vi "ClusterToBSONDocument.vi"(8 "error in (no error)":errorcluster, 11 "Variant":variant) -> (0 "error out":errorcluster, 3 "tBSONDocument out":refnum<class "tBSONDocument.lvclass">)   [LabVIEW 2013, in "BSON.lvlib" / "tBSONDocument.lvclass"]
doc: "Converts simple LabVIEW clusters into a BSON document. The cluster must contain only basic types including numerics, timestamps, strings, paths, booleans, and clusters. Single dimension arrays of these types are also supported. There is limited analog waveform support although waveform attributes are not added to the document."
uses:
  tBSONDocument.lvclass
  status.ctl
  addI32Element.vi
  addI64Element.vi
  addDoubleElement.vi
  addBooleanElement.vi
  addStringElement.vi
  addTimestampElement.vi
  addDocumentElement.vi
  addI32[]Element.vi
  addI64[]Element.vi
  addDouble[]Element.vi
  addBoolean[]Element.vi
  addString[]Element.vi
  addTimestamp[]Element.vi
  addDocument[]Element.vi
  <vilib>/Utility/VariantDataType/VariantType.lvlib
  BSON.lvlib
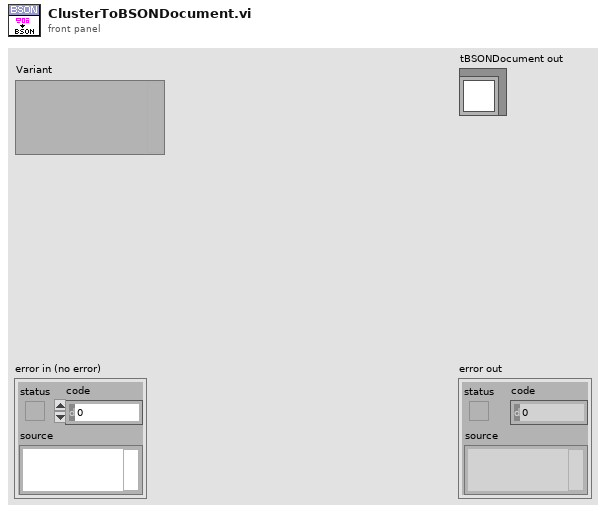
[diagram p1: front panel]
types:
  T1 = typedef "BSON.lvlib/status.ctl" = enum16{"Stream Corrupted or Ended Abruptly", "Incorrect Type In Stream", "ObjectID Invalid", "Method Not Implemented", "Invalid Name", "Invalid URI", "AutoReconnect", "Operation Failed", "Incorrectly Configured", "Cursor Not Found", "Timeout", "Invalid Type", "Empty Name", "Duplicate Name", "MD5Incorrect"}
  T2 = typedef "VariantType.lvlib/Type.ctl" = enum8{"Invalid Type", "Void", "I8", "I16", "I32", "I64", "U8", "U16", "U32", "U64", "Single Float", "Double Float", "Extended Float", "Single Complex", "Double Complex", "Extended Complex", "Enum U8", "Enum U16", "Enum U32", "Enum U64", "Single Float With Unit", "Double Float With Unit", "Extended Float With Unit", "Single Complex with Unit", "Double Complex with Unit", "Extended Complex with Unit", "Boolean", "String", "Path", "Picture", "Tag", "Array", "Cluster", "Variant", "LV Variant", "Waveform", "Timestamp", "Digital Waveform", "Digital Data", "ExpressData", "Refnum", "External Data", "VI", "Poly VI", "LabVIEW Class Instance", "Fixed Point"}
  T3 = typedef "VariantType.lvlib/MemoryInfo.ctl" = cluster{"Type":T4, "Size":u32}
  T4 = typedef "VariantType.lvlib/MemoryType.ctl" = enum16{"Variable", "Fixed", "Bounded"}
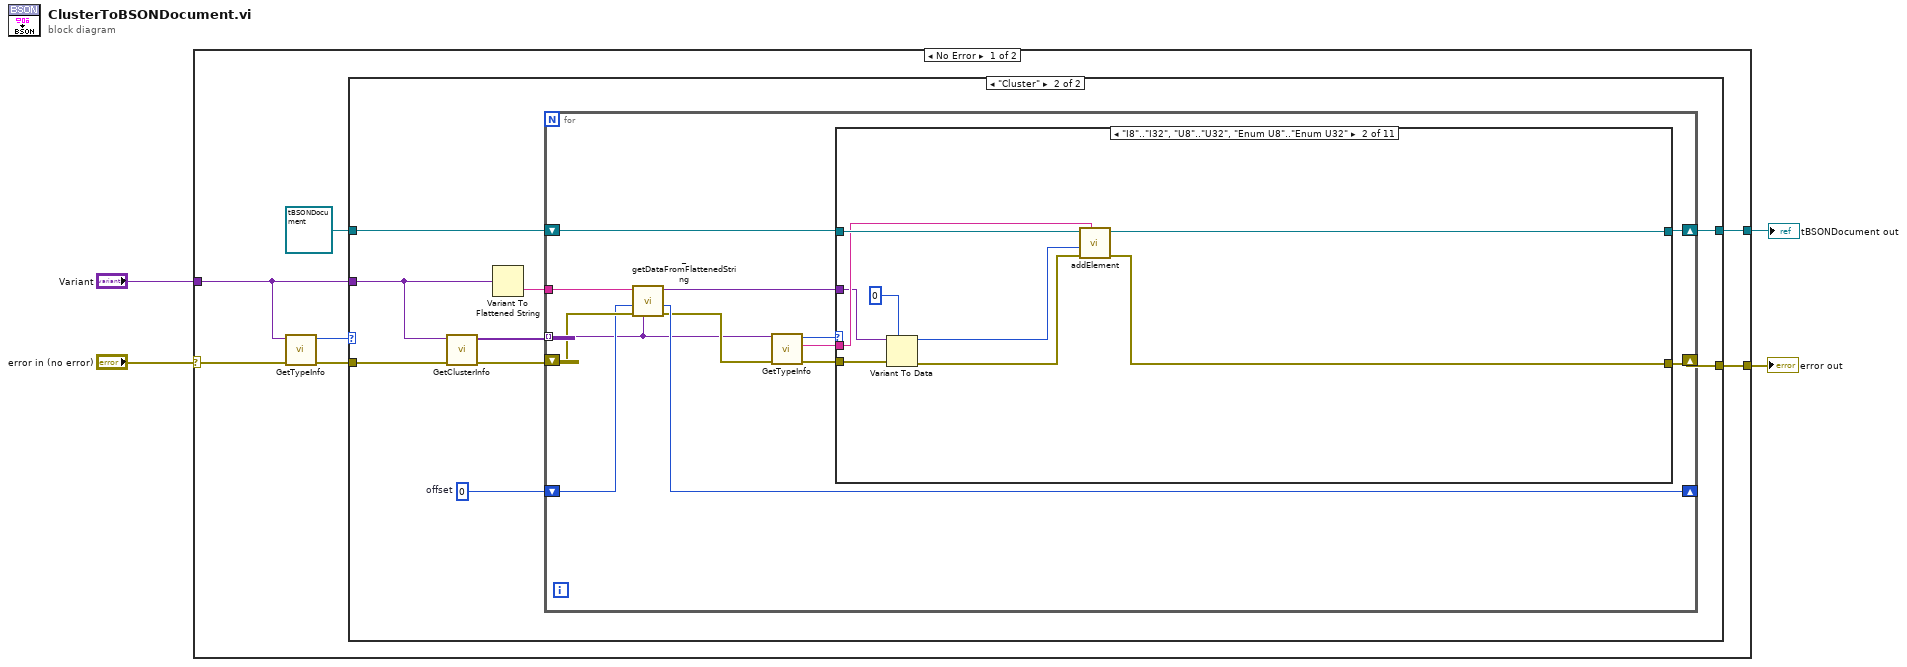
[diagram p0: block diagram]
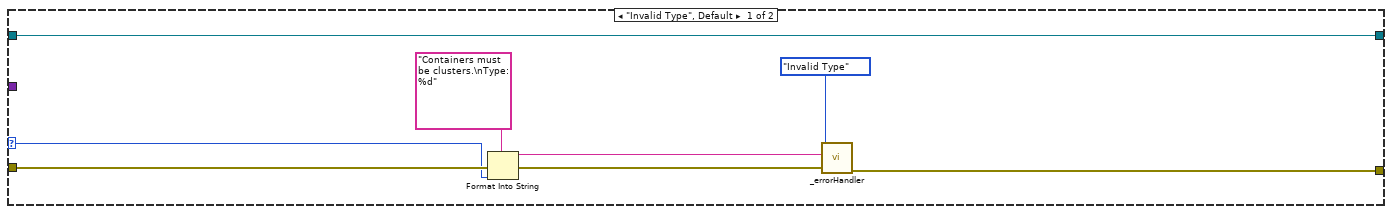
[diagram p2: hidden frame]
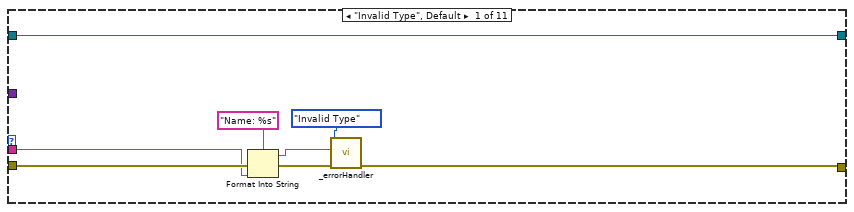
[diagram p3: hidden frame]
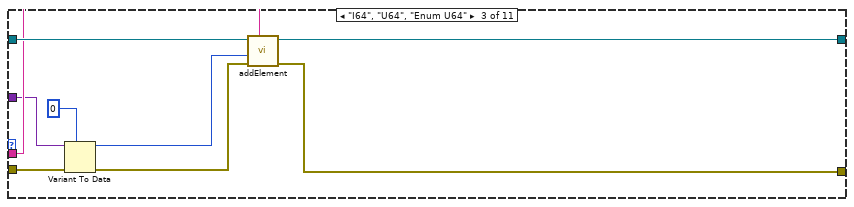
[diagram p4: hidden frame]
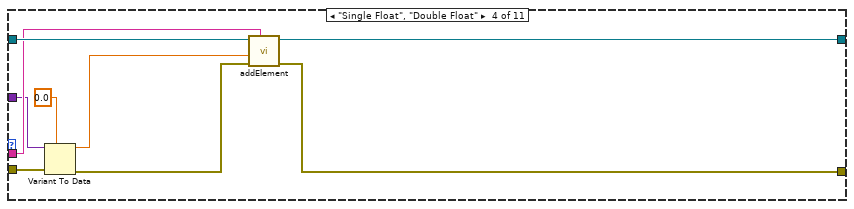
[diagram p5: hidden frame]
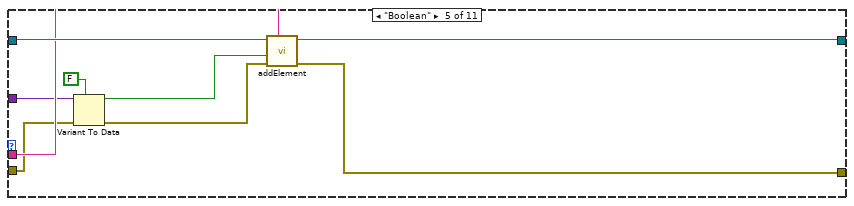
[diagram p6: hidden frame]
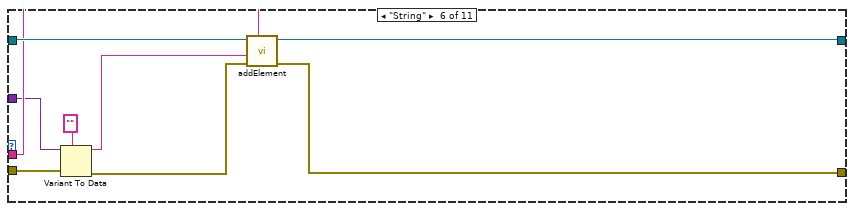
[diagram p7: hidden frame]
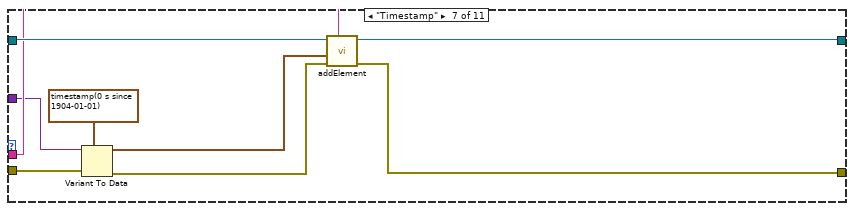
[diagram p8: hidden frame]
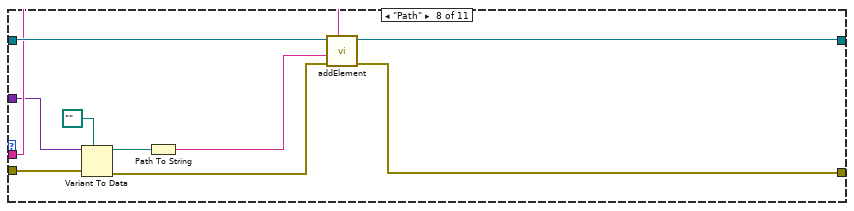
[diagram p9: hidden frame]
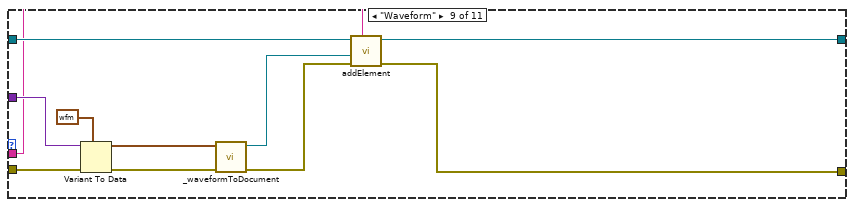
[diagram p10: hidden frame]
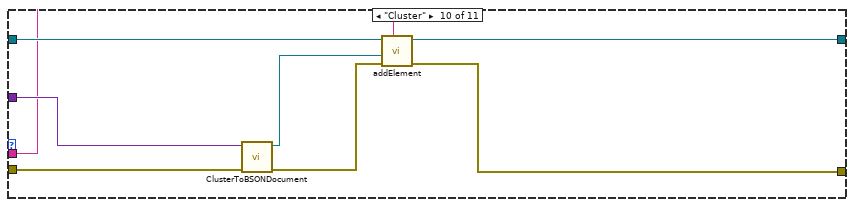
[diagram p11: hidden frame]
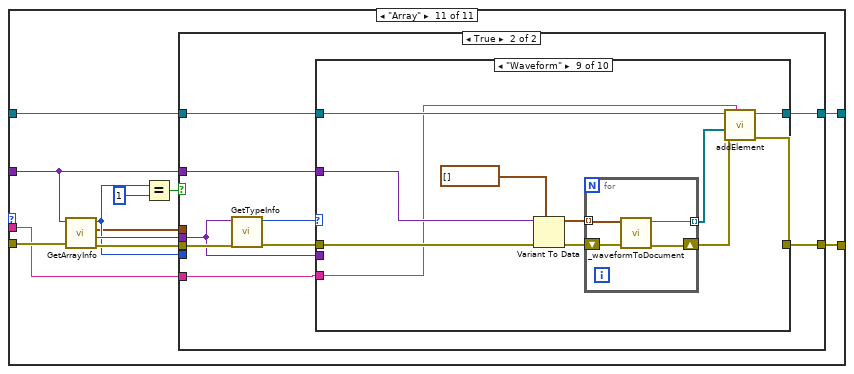
[diagram p12: hidden frame]
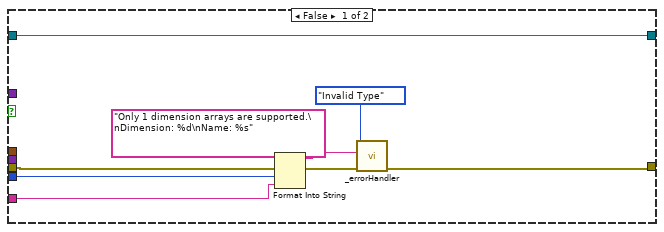
[diagram p13: hidden frame]
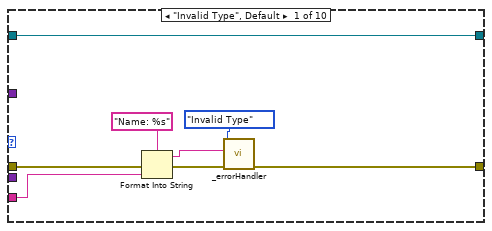
[diagram p14: hidden frame]
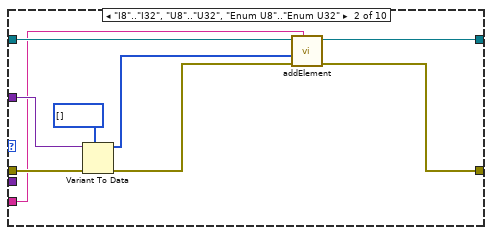
[diagram p15: hidden frame]
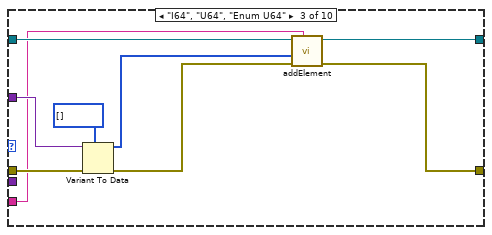
[diagram p16: hidden frame]
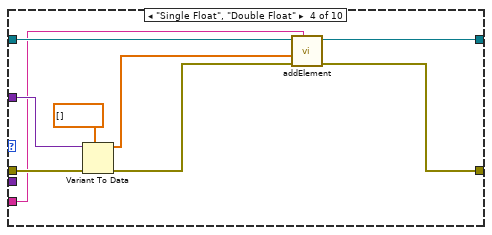
[diagram p17: hidden frame]
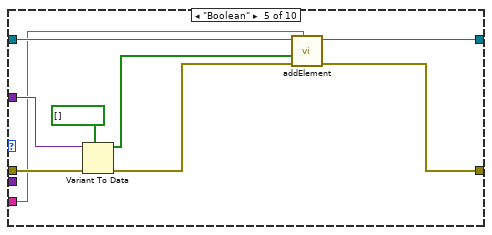
[diagram p18: hidden frame]
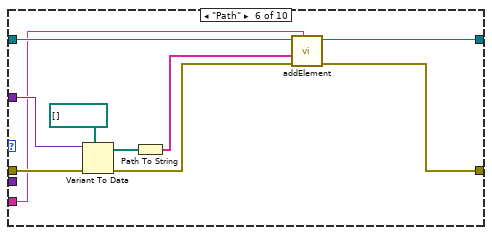
[diagram p19: hidden frame]
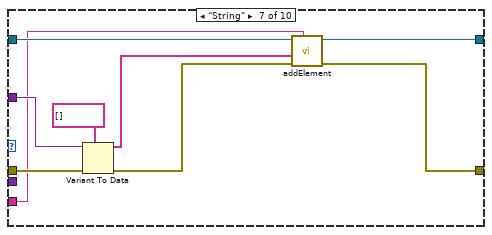
[diagram p20: hidden frame]
diagram:
  n1 = case shown="No Error" "error in (no error)" {
    selector: "error in (no error)" -> [w11 w266]
    tunnel: [w8 w266] -> w3
    tunnel: "Variant" -> [w7 _]
    tunnel: [w5 _] -> w2
    frame No Error {
      n2 = call <vilib>:"GetTypeInfo.vi"("error in (no error)"=w11, "Variant"=w7) -> ("error out"=w9:errorcluster, "Type Enum"=w10:T2)  [unwired: 5 in, 3 out]
      n3 = case shown="\"Cluster\"" w10 {
        selector: w10 -> [w12 _]
        tunnel: w9 -> [w18 w20]
        tunnel: [w14 w26] -> w8
        tunnel: w7 -> [_ w22]
        tunnel: refnum<class "tBSONDocument.lvclass"> refnum ("lvMongoDriver.lvlib:BSON.lvlib:tBSONDocument.lvclass") -> [w13 w27]
        tunnel: [w13 w24] -> w5
        frame "Invalid Type", Default {
          n4 = Format Into String(format string="Containers must be clusters.\nType: %d", error in=w18, w12) -> (resulting string=w15:string, error out=w17:errorcluster)  [unwired: 1 in]
          n5 = call "_errorHandler.vi"("error in (no error)"=w17, "Additional Text"=w15, "Error Type"=status."Invalid Type") -> ("error out"=w14:errorcluster)  [unwired: 8 in]
        }
        frame "Cluster" {
          w23 = 0  # offset
          n6 = call <vilib>:"GetClusterInfo.vi"("error in (no error)"=w20, "Variant"=w22) -> ("error out"=w28:errorcluster, "Cluster Elements"=w25:variant[])  [unwired: 8 in]
          n7 = Variant To Flattened String(Variant=w22) -> (data string=w21:string)  [unwired: 1 out]
          n8 = for {
            tunnel: w25 -> [w29] mode=indexing
            shift-right: [w38] -> w24
            shift-left: w27 -> [w41]
            shift-right: [w39] -> w26
            shift-left: w28 -> [w35]
            shift-right: [w33] -> _
            shift-left: w23 -> [w34]
            tunnel: w21 -> [w31]
            n9 = call "_getDataFromFlattenedString.vi"("type descriptor"=w29, "error in (no error)"=w35, "offset to extract data"=w34, "flattened data"=w31) -> ("error out"=w32:errorcluster, "offset past data"=w33:i32, "data"=w30:variant)  [unwired: 5 in]
            n10 = call <vilib>:"GetTypeInfo.vi"("error in (no error)"=w32, "Variant"=w29) -> ("error out"=w36:errorcluster, "Name"=w37:string, "Type Enum"=w40:T2)  [unwired: 5 in, 2 out]
            n11 = case shown="\"I8\"..\"I32\", \"U8\"..\"U32\", \"Enum U8\"..\"Enum U32\"" w40 {
              tunnel: w41 -> [w49 w57 w66 w76 w85 w93 w103 w113 w119 w130 w139]
              tunnel: [w47 w55 w61 w70 w82 w88 w98 w109 w117 w127 w140] -> w39
              tunnel: [w49 w54 w62 w75 w83 w89 w99 w110 w118 w126 w137] -> w38
              tunnel: w37 -> [w42 w52 w65 w74 w84 w90 w100 w111 w116 w125 w141]
              tunnel: w36 -> [w46 w51 w60 w69 w81 w87 w97 w108 w124 w131 w144]
              tunnel: w30 -> [_ w50 w59 w68 w80 w86 w96 w107 w123 w132 w138]
              frame "Invalid Type", Default {
                n12 = Format Into String(format string="Name: %s", error in=w46, w42) -> (resulting string=w44:string, error out=w45:errorcluster)  [unwired: 1 in]
                n13 = call "_errorHandler.vi"("error in (no error)"=w45, "Additional Text"=w44, "Error Type"=status."Invalid Type") -> ("error out"=w47:errorcluster)  [unwired: 8 in]
              }
              frame "I8".."I32", "U8".."U32", "Enum U8".."Enum U32" {
                n14 = Variant To Data(error in=w51, type=0, Variant=w50) -> (data=w53:i32, error out=w56:errorcluster)
                n15 = call-poly "addElement.vi"("Name"=w52, "error in (no error)"=w56, "Value"=w53, "tBSONDocument in"=w57) -> ("error out"=w55:errorcluster, "tBSONDocument out"=w54:refnum<class "tBSONDocument.lvclass">)  [unwired: 6 in]
              }
              frame "I64", "U64", "Enum U64" {
                n16 = Variant To Data(error in=w60, type=i64 0, Variant=w59) -> (data=w63:i64, error out=w64:errorcluster)
                n17 = call-poly "addElement.vi"("Name"=w65, "error in (no error)"=w64, "Value"=w63, "tBSONDocument in"=w66) -> ("error out"=w61:errorcluster, "tBSONDocument out"=w62:refnum<class "tBSONDocument.lvclass">)  [unwired: 6 in]
              }
              frame "Single Float", "Double Float" {
                n18 = Variant To Data(error in=w69, type=0.0, Variant=w68) -> (data=w72:dbl, error out=w71:errorcluster)
                n19 = call-poly "addElement.vi"("Name"=w74, "error in (no error)"=w71, "Value"=w72, "tBSONDocument in"=w76) -> ("error out"=w70:errorcluster, "tBSONDocument out"=w75:refnum<class "tBSONDocument.lvclass">)  [unwired: 6 in]
              }
              frame "Boolean" {
                n20 = Variant To Data(error in=w81, type=FALSE, Variant=w80) -> (data=w79:bool, error out=w78:errorcluster)
                n21 = call-poly "addElement.vi"("Name"=w84, "error in (no error)"=w78, "Value"=w79, "tBSONDocument in"=w85) -> ("error out"=w82:errorcluster, "tBSONDocument out"=w83:refnum<class "tBSONDocument.lvclass">)  [unwired: 6 in]
              }
              frame "String" {
                n22 = Variant To Data(error in=w87, type="", Variant=w86) -> (data=w91:string, error out=w92:errorcluster)
                n23 = call-poly "addElement.vi"("Name"=w90, "error in (no error)"=w92, "Value"=w91, "tBSONDocument in"=w93) -> ("error out"=w88:errorcluster, "tBSONDocument out"=w89:refnum<class "tBSONDocument.lvclass">)  [unwired: 6 in]
              }
              frame "Timestamp" {
                n24 = Variant To Data(error in=w97, type=timestamp(0 s since 1904-01-01), Variant=w96) -> (data=w101:timestamp, error out=w102:errorcluster)
                n25 = call-poly "addElement.vi"("Name"=w100, "error in (no error)"=w102, "Value"=w101, "tBSONDocument in"=w103) -> ("error out"=w98:errorcluster, "tBSONDocument out"=w99:refnum<class "tBSONDocument.lvclass">)  [unwired: 6 in]
              }
              frame "Path" {
                n26 = Variant To Data(error in=w108, type=path "", Variant=w107) -> (data=w105:path, error out=w112:errorcluster)
                n27 = Path To String(path=w105) -> (string=w104:string)
                n28 = call-poly "addElement.vi"("Name"=w111, "error in (no error)"=w112, "Value"=w104, "tBSONDocument in"=w113) -> ("error out"=w109:errorcluster, "tBSONDocument out"=w110:refnum<class "tBSONDocument.lvclass">)  [unwired: 6 in]
              }
              frame "Waveform" {
                n29 = Variant To Data(error in=w124, type=waveform(dbl) {"t0"=timestamp(0 s since 1904-01-01), "dt"=1.0, "Y"=[]} ("waveform"), Variant=w123) -> (data=w121:waveform(dbl), error out=w120:errorcluster)
                n30 = call "_waveformToDocument.vi"("error in (no error)"=w120, "waveform"=w121) -> ("error out"=w114:errorcluster, "tBSONDocument out"=w115:refnum<class "tBSONDocument.lvclass">)  [unwired: 8 in]
                n31 = call-poly "addElement.vi"("Name"=w116, "error in (no error)"=w114, "Value"=w115, "tBSONDocument in"=w119) -> ("error out"=w117:errorcluster, "tBSONDocument out"=w118:refnum<class "tBSONDocument.lvclass">)  [unwired: 6 in]
              }
              frame "Cluster" {
                n32 = call "ClusterToBSONDocument.vi"("error in (no error)"=w131, "Variant"=w132) -> ("error out"=w128:errorcluster, "tBSONDocument out"=w129:refnum<class "tBSONDocument.lvclass">)  [unwired: 8 in]
                n33 = call-poly "addElement.vi"("Name"=w125, "error in (no error)"=w128, "Value"=w129, "tBSONDocument in"=w130) -> ("error out"=w127:errorcluster, "tBSONDocument out"=w126:refnum<class "tBSONDocument.lvclass">)  [unwired: 6 in]
              }
              frame "Array" {
                n34 = call <vilib>:"GetArrayInfo.vi"("error in (no error)"=w144, "Variant"=w138) -> ("error out"=w143:errorcluster, "ArrayElement"=w142:variant, "Array Lengths"=w133:T3[], "NDims"=w136:i32)  [unwired: 6 in]
                n35 = Equal?(x=w136, y=1) -> (x = y?=w134:bool)
                n36 = case shown="True" w134 {
                  tunnel: w143 -> [w149 w162]
                  tunnel: w142 -> [_ w155]
                  tunnel: w141 -> [w148 w159]
                  tunnel: [w146 w158] -> w140
                  tunnel: w139 -> [w145 w157]
                  tunnel: w138 -> [_ w156]
                  tunnel: w136 -> [w147 _]
                  tunnel: [w145 w154] -> w137
                  tunnel: w133 -> [_ _]
                  frame False {
                    n37 = Format Into String(format string="Only 1 dimension arrays are supported.\nDimension: %d\nName: %s", error in=w149, w147, w148) -> (resulting string=w151:string, error out=w152:errorcluster)  [unwired: 1 in]
                    n38 = call "_errorHandler.vi"("error in (no error)"=w152, "Additional Text"=w151, "Error Type"=status."Invalid Type") -> ("error out"=w146:errorcluster)  [unwired: 8 in]
                  }
                  frame True {
                    n39 = call <vilib>:"GetTypeInfo.vi"("error in (no error)"=w162, "Variant"=w155) -> ("error out"=w161:errorcluster, "Type Enum"=w160:T2)  [unwired: 5 in, 3 out]
                    n40 = case shown="\"Waveform\"" w160 {
                      tunnel: w161 -> [w166 w179 w188 w197 w206 w216 w225 w234 w245 w255]
                      tunnel: w159 -> [w165 w171 w180 w189 w198 w209 w217 w226 w239 w256]
                      tunnel: [w164 w173 w182 w191 w200 w211 w219 w228 w241 w258] -> w158
                      tunnel: w157 -> [w163 w176 w185 w194 w203 w213 w222 w231 w242 w261]
                      tunnel: w156 -> [_ w178 w187 w196 w205 w215 w224 w233 w244 w254]
                      tunnel: [w163 w172 w181 w190 w199 w210 w218 w227 w240 w257] -> w154
                      tunnel: w155 -> [_ _ _ _ _ _ _ _ _ w253]
                      frame "Invalid Type", Default {
                        n41 = Format Into String(format string="Name: %s", error in=w166, w165) -> (resulting string=w168:string, error out=w169:errorcluster)  [unwired: 1 in]
                        n42 = call "_errorHandler.vi"("error in (no error)"=w169, "Additional Text"=w168, "Error Type"=status."Invalid Type") -> ("error out"=w164:errorcluster)  [unwired: 8 in]
                      }
                      frame "I8".."I32", "U8".."U32", "Enum U8".."Enum U32" {
                        n43 = Variant To Data(error in=w179, type=i32[] [], Variant=w178) -> (data=w174:i32[], error out=w175:errorcluster)
                        n44 = call-poly "addElement.vi"("Name"=w171, "error in (no error)"=w175, "Value"=w174, "tBSONDocument in"=w176) -> ("error out"=w173:errorcluster, "tBSONDocument out"=w172:refnum<class "tBSONDocument.lvclass">)  [unwired: 6 in]
                      }
                      frame "I64", "U64", "Enum U64" {
                        n45 = Variant To Data(error in=w188, type=i64[] [], Variant=w187) -> (data=w183:i64[], error out=w184:errorcluster)
                        n46 = call-poly "addElement.vi"("Name"=w180, "error in (no error)"=w184, "Value"=w183, "tBSONDocument in"=w185) -> ("error out"=w182:errorcluster, "tBSONDocument out"=w181:refnum<class "tBSONDocument.lvclass">)  [unwired: 6 in]
                      }
                      frame "Single Float", "Double Float" {
                        n47 = Variant To Data(error in=w197, type=dbl[] [], Variant=w196) -> (data=w192:dbl[], error out=w193:errorcluster)
                        n48 = call-poly "addElement.vi"("Name"=w189, "error in (no error)"=w193, "Value"=w192, "tBSONDocument in"=w194) -> ("error out"=w191:errorcluster, "tBSONDocument out"=w190:refnum<class "tBSONDocument.lvclass">)  [unwired: 6 in]
                      }
                      frame "Boolean" {
                        n49 = Variant To Data(error in=w206, type=bool[] [], Variant=w205) -> (data=w201:bool[], error out=w202:errorcluster)
                        n50 = call-poly "addElement.vi"("Name"=w198, "error in (no error)"=w202, "Value"=w201, "tBSONDocument in"=w203) -> ("error out"=w200:errorcluster, "tBSONDocument out"=w199:refnum<class "tBSONDocument.lvclass">)  [unwired: 6 in]
                      }
                      frame "Path" {
                        n51 = Variant To Data(error in=w216, type=path[] [], Variant=w215) -> (data=w208:path[], error out=w212:errorcluster)
                        n52 = Path To String(path=w208) -> (string=w207:string[])
                        n53 = call-poly "addElement.vi"("Name"=w209, "error in (no error)"=w212, "Value"=w207, "tBSONDocument in"=w213) -> ("error out"=w211:errorcluster, "tBSONDocument out"=w210:refnum<class "tBSONDocument.lvclass">)  [unwired: 6 in]
                      }
                      frame "String" {
                        n54 = Variant To Data(error in=w225, type=string[] [], Variant=w224) -> (data=w220:string[], error out=w221:errorcluster)
                        n55 = call-poly "addElement.vi"("Name"=w217, "error in (no error)"=w221, "Value"=w220, "tBSONDocument in"=w222) -> ("error out"=w219:errorcluster, "tBSONDocument out"=w218:refnum<class "tBSONDocument.lvclass">)  [unwired: 6 in]
                      }
                      frame "Timestamp" {
                        n56 = Variant To Data(error in=w234, type=timestamp[] [], Variant=w233) -> (data=w229:timestamp[], error out=w230:errorcluster)
                        n57 = call-poly "addElement.vi"("Name"=w226, "error in (no error)"=w230, "Value"=w229, "tBSONDocument in"=w231) -> ("error out"=w228:errorcluster, "tBSONDocument out"=w227:refnum<class "tBSONDocument.lvclass">)  [unwired: 6 in]
                      }
                      frame "Waveform" {
                        n58 = Variant To Data(error in=w245, type=waveform(dbl)[] [], Variant=w244) -> (data=w237:waveform(dbl)[], error out=w238:errorcluster)
                        n59 = for {
                          shift-right: [w247] -> w235
                          shift-left: w238 -> [w249]
                          tunnel: w237 -> [w248] mode=indexing
                          tunnel: [w246] -> w236 mode=indexing
                          n60 = call "_waveformToDocument.vi"("error in (no error)"=w249, "waveform"=w248) -> ("error out"=w247:errorcluster, "tBSONDocument out"=w246:refnum<class "tBSONDocument.lvclass">)  [unwired: 8 in]
                        }
                        n61 = call-poly "addElement.vi"("Name"=w239, "error in (no error)"=w235, "Value"=w236, "tBSONDocument in"=w242) -> ("error out"=w241:errorcluster, "tBSONDocument out"=w240:refnum<class "tBSONDocument.lvclass">)  [unwired: 6 in]
                      }
                      frame "Cluster" {
                        n62 = Build Array(w253) -> (w252:variant[])
                        n63 = Variant To Data(error in=w255, type=w252, Variant=w254) -> (data=w251:variant[], error out=w250:errorcluster)
                        n64 = for {
                          shift-right: [w265] -> w259
                          shift-left: w250 -> [w262]
                          tunnel: [w264] -> w260 mode=indexing
                          tunnel: w251 -> [w263] mode=indexing
                          n65 = call "ClusterToBSONDocument.vi"("error in (no error)"=w262, "Variant"=w263) -> ("error out"=w265:errorcluster, "tBSONDocument out"=w264:refnum<class "tBSONDocument.lvclass">)  [unwired: 8 in]
                        }
                        n66 = call-poly "addElement.vi"("Name"=w256, "error in (no error)"=w259, "Value"=w260, "tBSONDocument in"=w261) -> ("error out"=w258:errorcluster, "tBSONDocument out"=w257:refnum<class "tBSONDocument.lvclass">)  [unwired: 6 in]
                      }
                    }
                  }
                }
              }
            }
          }
        }
      }
    }
    frame Error {
    }
  }
  "error out" <- w3
  "tBSONDocument out" <- w2
